vi "RTheta_SubVI.vi"(9 "B":dbl, 10 "SR":dbl, 11 "SL":dbl) -> (2 "Theta":dbl, 3 "R":dbl)   [LabVIEW 2017]
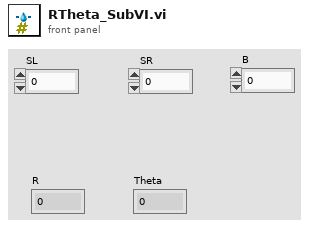
[diagram p1: front panel]
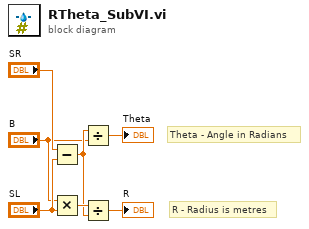
[diagram p0: block diagram]
diagram:
  # "R - Radius is metres"
  # "Theta - Angle in Radians"
  n1 = Subtract(x="SR", y="SL") -> (x-y=w3:dbl)
  n2 = Multiply(x="B", y="SL") -> (x*y=w6:dbl)
  n3 = Divide(x=w3, y="B") -> (x/y=→"Theta":dbl)
  n4 = Divide(x=w6, y=w3) -> (x/y=→"R":dbl)
